vi "FTW-TransferClient-Upload.vi"(0 "Transfer Client":refnum<class "FTW-TransferClient-dotNET.lvclass">, 5 "Data":string, 7 "Remote Filename":string, 11 "error in":errorcluster) -> (4 "Transfer Client out":refnum<class "FTW-TransferClient-dotNET.lvclass">, 6 "URI":string, 8 "Response":string, 10 "Upload Time":u32 format="%06dmsec", 15 "error out":errorcluster)   [LabVIEW 2015, in "FTW-TransferClient-dotNET.lvclass"]
uses:
  FTW-TransferClient-dotNET.lvclass
  FTW-TransferClient-dotNET.lvclass/FTW-TransferClient-dotNET.ctl
panel:
  # "Inputs"
  # "Outputs"
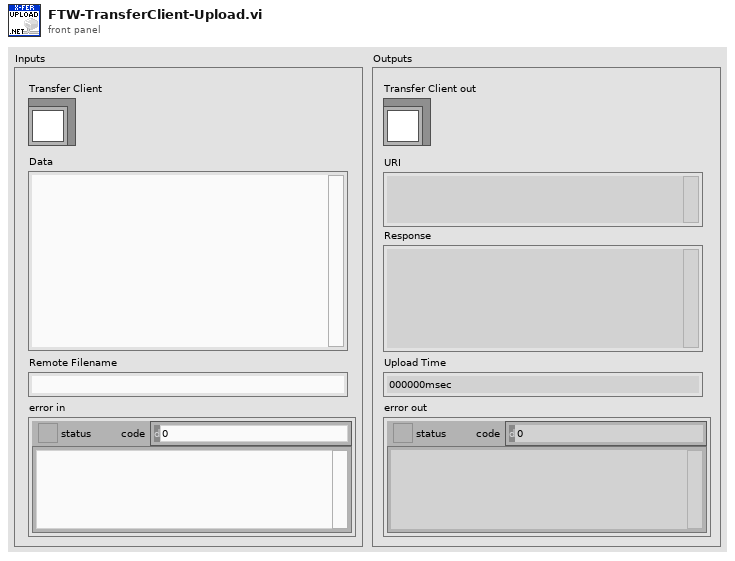
[diagram p1: front panel]
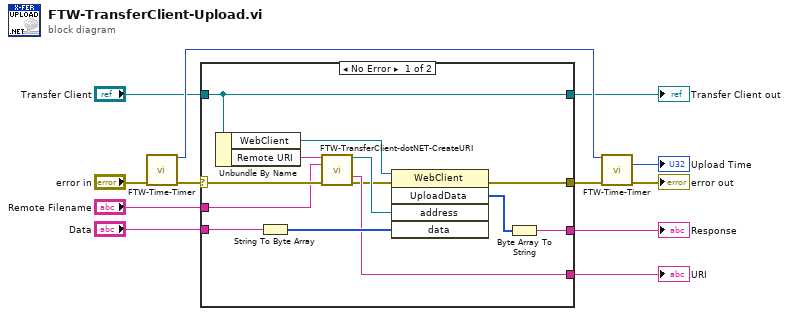
[diagram p0: block diagram]
diagram:
  n1 = call "FTW-Time-Timer.vi"("error in"="error in") -> ("Current Tick Count"=w10:u32, "error out"=w12:errorcluster)  [unwired: 12 in, 1 out]
  n2 = case shown="No Error" w12 {
    selector: w12 -> [w14 w26]
    tunnel: "Transfer Client" -> [w22 w27]
    tunnel: [w25 _] -> w7
    tunnel: [w24 w26] -> w11
    tunnel: [w22 w27] -> w8
    tunnel: [w16 _] -> w6
    tunnel: "Data" -> [w20 _]
    tunnel: "Remote Filename" -> [w13 _]
    frame No Error {
      n3 = Unbundle By Name(w22) -> ("WebClient"=w23:refnum<k24>, "Remote URI"=w18:string)
      n4 = String To Byte Array(string=w20) -> (unsigned byte array=w19:u8[])
      n5 = call "FTW-TransferClient-dotNET-CreateURI.vi"("URI"=w18, "Relative URI"=w13, "error in"=w14) -> ("URI ref"=w17:refnum<k24>, "AbsoluteURI"=w16:string, "error out"=w15:errorcluster)  [unwired: 7 in, 3 out]
      n6 = invoke class="WebClient" method="UploadData"(reference=w23, error in=w15, "address"=w17, "data"=w19) -> (error out=w24:errorcluster, "UploadData"=w21:u8[])  [unwired: 1 in, 3 out]
      n7 = Byte Array To String(unsigned byte array=w21) -> (string=w25:string)
    }
    frame Error {
    }
  }
  "Transfer Client out" <- w8
  "URI" <- w6
  "Response" <- w7
  n8 = call "FTW-Time-Timer.vi"("Initial Tick Count"=w10, "error in"=w11) -> ("Elapsed Time"=→"Upload Time":u32, "error out"=→"error out":errorcluster)  [unwired: 11 in, 1 out]
